vi "convert To Velocity.vi"(10 "gearRatio":sgl, 11 "velVal":i16) -> (3 "function return":sgl)   [LabVIEW 2023, in "SADI_FW3.lvlib"]
doc: "SADI_API_Wrapper float convertToVelocity(int16_t velVal,float gearRatio);"
uses:
  SADI_FW3.lvlib
  SADI_FW3.dll
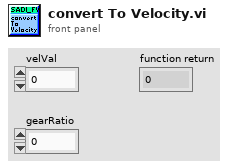
[diagram p1: front panel]
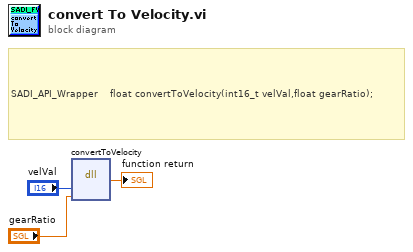
[diagram p0: block diagram]
diagram:
  # "SADI_API_Wrapper    float convertToVelocity(int16_t velVal,float gearRatio);"
  n1 = dll-call lib="C:/Users/loran/Documents/School/24_Spring/Controls Lab/EML4314c_Sp24_framework_0/LVLib/SADI_FW3.*" fn="convertToVelocity"("velVal"="velVal", "gearRatio"="gearRatio") -> (→"function return":sgl)  [unwired: 5 in, 2 out]
